vi "Display Text.vi"(0 "Refnum in":refnum<k20>, 1 "Brightness":u8=1 min=1 step=1, 2 "Font, Size & Style":T1={"Desired Font (Application)"=enum."Application Font", "[User-specified Font]"={"Font Name"="", "Size"=12, "Strikeout?"=FALSE, "Italic?"=FALSE, "Underline?"=FALSE, "Outline?"=FALSE, "Shadow?"=FALSE, "Bold?"=FALSE, "Rotation Angle"=0.0}, "Horizontal Alignment"=0, "Vertical Alignment"=0} {"Vertical Alignment" items=["Bottom", "Top", "Baseline"]; "Horizontal Alignment" items=["Left", "Center", "Right"]; "[User-specified Font]"."Rotation Angle" format="%.2f"}, 5 "String":string, 9 "Origin":cluster{"X":i32, "Y":i32}, 11 "error in (no error)":errorcluster, 12 "Text Color":u32(colorbox)=16777215, 13 "Text BG Color":u32(colorbox), 14 "Rect BG Color":u32(colorbox)) -> (3 "LED Matrix":picture, 4 "Refnum out":refnum<k20>, 15 "error out":errorcluster)   [LabVIEW 2013]
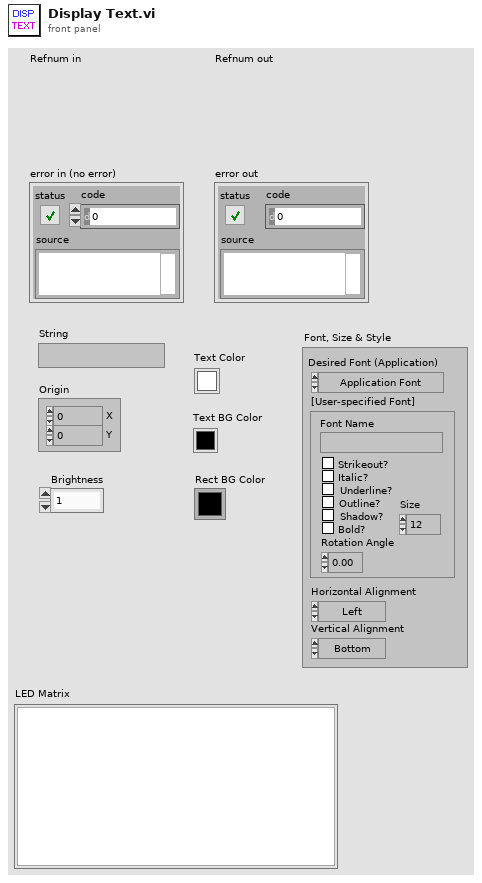
[diagram p1: front panel]
types:
  T1 = cluster{"Desired Font (Application)":enum16{"User-specified Font", "Application Font", "System Font", "Dialog Font"}, "[User-specified Font]":cluster{"Font Name":string, "Size":i16, "Strikeout?":bool, "Italic?":bool, "Underline?":bool, "Outline?":bool, "Shadow?":bool, "Bold?":bool, "Rotation Angle":dbl}, "Horizontal Alignment":i16, "Vertical Alignment":i16}
  T2 = cluster{"Left":i32, "Top":i32, "Right":i32, "Bottom":i32}
  T3 = typedef "Image Type" = u32
  T4 = typedef "IMAQ Image.ctl" = refnum<image>
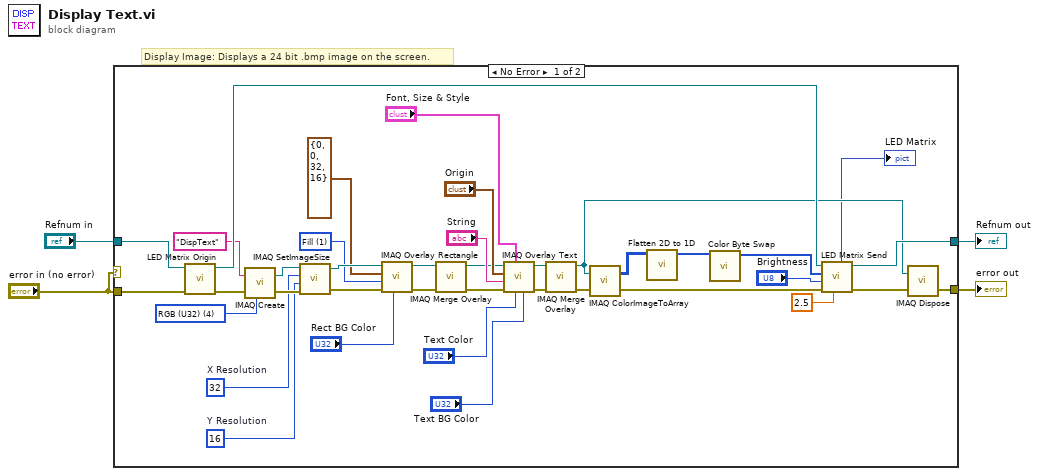
[diagram p0: block diagram]
diagram:
  # "Display Image: Displays a 24 bit .bmp image on the screen."
  n1 = case shown="No Error" "error in (no error)" {
    tunnel: "error in (no error)" -> [w41 w43]
    tunnel: "Refnum in" -> [w42 w44]
    tunnel: [w32 w43] -> w3
    tunnel: [w38 w44] -> w2
    frame No Error {
      w18 = u32 1 items=["Frame", "Fill", "Highlight"] ("Drawing Mode (Frame)")
      w23 = 16  # Y Resolution
      w24 = 32  # X Resolution
      w30 = T3 4 items=["Grayscale (U8)", "Grayscale (I16)", "Grayscale (SGL)", "Complex (CSG)", "RGB (U32)", "HSL (U32)", "RGB (U64)", "Grayscale (U16)"] ("Image Type")
      n2 = call "LED Matrix Origin.vi"("error in (no error)"=w41, "Refnum in"=w42) -> ("error out"=w31:errorcluster, "Refnum out"=w40:refnum<k20>)  [unwired: 8 in]
      n3 = call "IMAQ Create"("Image Name"="DispText", "Image Type"=w30, "error in (no error)"=w31) -> ("New Image"=w26:T4, "error out"=w25:errorcluster)  [unwired: 2 in]
      n4 = call "IMAQ SetImageSize"("error in (no error)"=w25, "Y Resolution"=w23, "X Resolution"=w24, "Image"=w26) -> ("error out"=w19:errorcluster, "Image Out"=w20:T4)  [unwired: 1 in]
      n5 = call "IMAQ Overlay Rectangle"("Color"="Rect BG Color", "error in (no error)"=w19, "Drawing Mode (Frame)"=w18, "Rectangle"=T2 {"Left"=0, "Top"=0, "Right"=32, "Bottom"=16}, "Image"=w20) -> ("error out"=w10:errorcluster, "Image Out"=w9:T4)  [unwired: 5 in]
      n6 = call "IMAQ Merge Overlay"("error in (no error)"=w10, "Image Src"=w9) -> ("error out"=w7:errorcluster, "Image Dst Out"=w8:T4)  [unwired: 8 in]
      n7 = call "IMAQ Overlay Text"("BG Color (Transparent)"="Text BG Color", "Text Color (black)"="Text Color", "Font, Size & Style"="Font, Size & Style", "error in (no error)"=w7, "String"="String", "Origin"="Origin", "Image"=w8) -> ("error out"=w14:errorcluster, "Image Out"=w15:T4)  [unwired: 3 in]
      n8 = call "IMAQ Merge Overlay"("error in (no error)"=w14, "Image Src"=w15) -> ("error out"=w13:errorcluster, "Image Dst Out"=w12:T4)  [unwired: 8 in]
      n9 = call "IMAQ ColorImageToArray"("Image"=w12, "error in (no error)"=w13) -> ("Image Pixels (U32)"=w28:u32[][], "error out"=w11:errorcluster)  [unwired: 2 in, 1 out]
      n10 = call "Flatten 2D to 1D.vi"("Image Pixels (U32) in"=w28) -> ("Image Pixels (U32) out"=w22:u32[])  [unwired: 10 in]
      n11 = call "Color Byte Swap.vi"("Image Pixels (U32) in"=w22) -> ("Images Pixels Out"=w21:u32[])  [unwired: 10 in]
      n12 = call "LED Matrix Send.vi"("Gamma"=2.5 ("Factor"), "error in (no error)"=w11, "Brightness"="Brightness", "Data"=w21, "Refnum in"=w40) -> ("error out"=w33:errorcluster, "Refnum out"=w38:refnum<k20>, "LED Matrix"=→"LED Matrix":picture)  [unwired: 3 in]
      n13 = call "IMAQ Dispose"("Image"=w12, "error in (no error)"=w33) -> ("error out"=w32:errorcluster)  [unwired: 4 in]
    }
    frame Error {
    }
  }
  "error out" <- w3
  "Refnum out" <- w2
